vi "Scalar Destroy (Polymorphic).vi"   [LabVIEW 2010]
uses:
  <vilib>/MDSplus/Library/MDSplus.lvlib
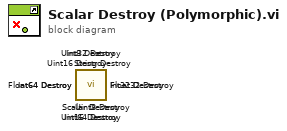
[diagram p0: block diagram]
diagram:
  n1 = call <vilib>:"Scalar Destroy.vi"() -> ()  [unwired: 11 in, 1 out]
  n2 = call <vilib>:"String Destroy.vi"() -> ()  [unwired: 11 in, 1 out]
  n3 = call <vilib>:"Float64 Destroy.vi"() -> ()  [unwired: 11 in, 1 out]
  n4 = call <vilib>:"Float32 Destroy.vi"() -> ()  [unwired: 11 in, 1 out]
  n5 = call <vilib>:"Uint64 Destroy.vi"() -> ()  [unwired: 11 in, 1 out]
  n6 = call <vilib>:"Uint32 Destroy.vi"() -> ()  [unwired: 11 in, 1 out]
  n7 = call <vilib>:"Uint16 Destroy.vi"() -> ()  [unwired: 11 in, 1 out]
  n8 = call <vilib>:"Uint8 Destroy.vi"() -> ()  [unwired: 11 in, 1 out]
  n9 = call <vilib>:"Int64 Destroy.vi"() -> ()  [unwired: 11 in, 1 out]
  n10 = call <vilib>:"Int32 Destroy.vi"() -> ()  [unwired: 11 in, 1 out]
  n11 = call <vilib>:"Int16 Destroy.vi"() -> ()  [unwired: 11 in, 1 out]
  n12 = call <vilib>:"Int8 Destroy.vi"() -> ()  [unwired: 11 in, 1 out]
